vi "SetWavelength.vi"(8 "error in (no error)":errorcluster, 10 "Wavelength":dbl format="%#_13g", 11 "OPM in":refnum<class "OPM.lvclass">) -> (0 "error out":errorcluster, 3 "OPM out":refnum<class "OPM.lvclass">)   [LabVIEW 2017, in "OPM.lvclass"]
uses:
  OPM.lvclass
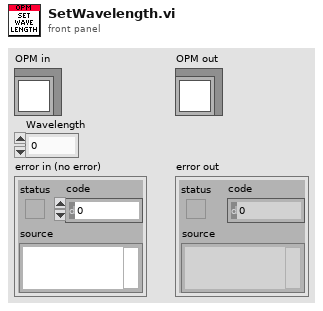
[diagram p1: front panel]
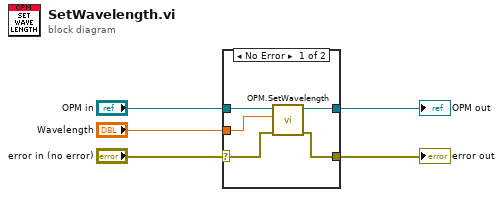
[diagram p0: block diagram]
diagram:
  n1 = case shown="No Error" "error in (no error)" {
    selector: "error in (no error)" -> [w8 w12]
    tunnel: [w7 w12] -> w4
    tunnel: [w6 w11] -> w2
    tunnel: "OPM in" -> [w10 w11]
    tunnel: "Wavelength" -> [w9 _]
    frame No Error {
      n2 = call-dynamic "OPM.SetWavelength.vi"("error in (no error)"=w8, "Wavelength, nm"=w9, "OPM in"=w10) -> ("error out"=w7:errorcluster, "OPM out"=w6:refnum<class "OPM.lvclass">)  [unwired: 7 in]
    }
    frame Error {
    }
  }
  "error out" <- w4
  "OPM out" <- w2
